vi "Create Resources.vi"   [LabVIEW 2015, in "niInstr AXI4-Lite Address Space Collection v1 FPGA.lvclass"]
doc: "Creates a new FPGA resource of the selected type.\n\n<b>Do not place this VI into a case structure or it will not compile correctly!</b>"
uses:
  <instrlib>/_niInstr/CLIP Adapters/v1/FPGA/AXI4-Lite/Address Space Collection/niInstr AXI4-Lite Address Space Collection v1 FPGA.lvclass
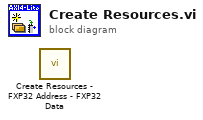
[diagram p0: block diagram]
diagram:
  n1 = call <instrlib>:"Create Resources - FXP32 Address - FXP32 Data.vi"() -> ()  [unwired: 15 in, 1 out]
